vi "Tools_System CPU Usage.vi"(8 "error in":errorcluster, 11 "CPU Usage Ref":T1) -> (0 "error out":errorcluster, 2 "CPU Usage (%)":dbl, 3 "CPU Usage Ref":T1)   [LabVIEW 2015, in "Performance.lvlib"]
doc: "Read the current CPU Usage. This VI should not be called more than once a second to allow for adequate averaging in the CPU Usage value."
uses:
  Performance.lvlib
  pdh.dll
  tools_system CPU Usage Ref.ctl
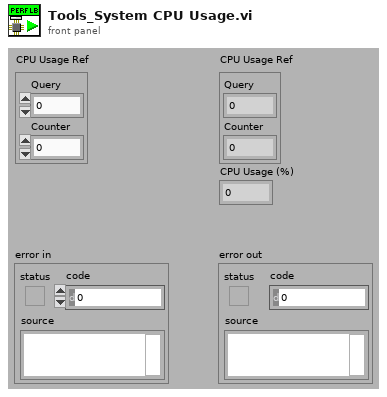
[diagram p1: front panel]
types:
  T1 = typedef "Performance.lvlib/tools_system CPU Usage Ref.ctl" = cluster{"Query":u32, "Counter":u32}
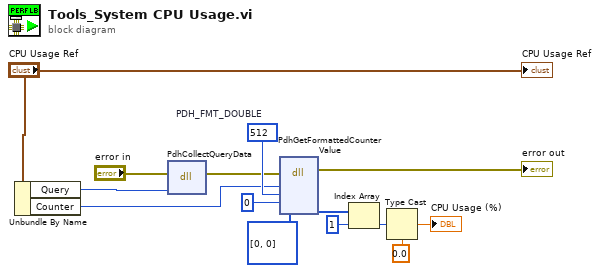
[diagram p0: block diagram]
diagram:
  w13 = u32 512  # PDH_FMT_DOUBLE
  n1 = Unbundle By Name("CPU Usage Ref") -> ("Query"=w2:u32, "Counter"=w1:u32)
  n2 = dll-call lib="pdh.dll" fn="PdhCollectQueryData"(error in="error in", "hQuery"=w2) -> (error out=w5:errorcluster)  [unwired: 4 in, 1 out]
  n3 = dll-call lib="pdh.dll" fn="PdhGetFormattedCounterValue"(error in=w5, "hCounter"=w1, "dwFormat"=w13, "lpdwType"=u32 0, "pValue"=u64[] [0, 0]) -> (error out=→"error out":errorcluster, "pValue"=w14:u64[])  [unwired: 6 in, 1 out]
  n4 = Index Array(array=w14, index=1) -> (element=w7:u64)
  n5 = Type Cast(type=0.0, x=w7) -> (*(type *) &x=→"CPU Usage (%)":dbl)
  "CPU Usage Ref" <- "CPU Usage Ref"
